vi "GS_Read_Config.vi"(4 "error in (no error)":errorcluster, 7 "Config Refnum":T1) -> (0 "error out":errorcluster, 2 "All Found?":bool, 3 "refnum out":T1)   [LabVIEW 2015]
uses:
  <vilib>/Utility/config.llb/Config Data RefNum.ctl
  <vilib>/Utility/config.llb/Read Key (Double).vi
  GSCS Scripting/Utils/GSP_Wavelength_Global.vi
  <vilib>/Utility/config.llb/NI_LVConfig.lvlib
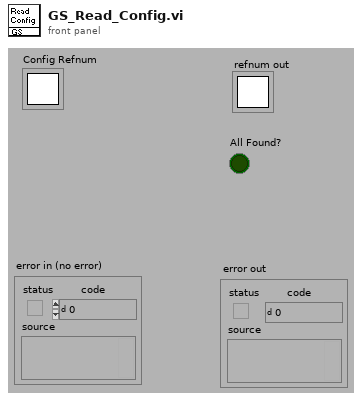
[diagram p1: front panel]
types:
  T1 = typedef "NI_LVConfig.lvlib/Config Data RefNum.ctl" = refnum<k1>
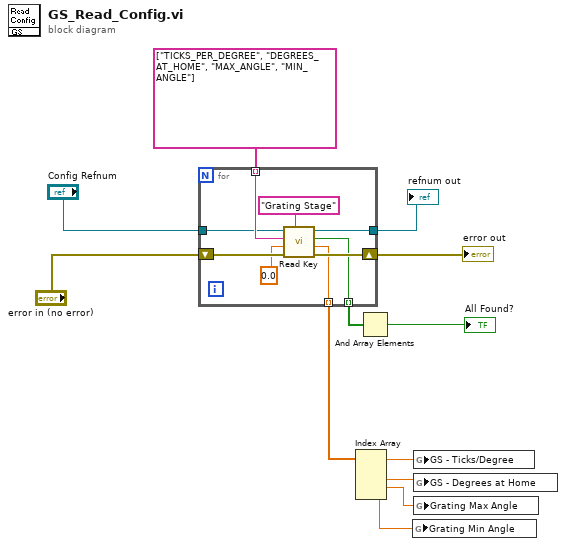
[diagram p0: block diagram]
diagram:
  n1 = for {
    shift-right: [w19] -> w11
    shift-left: "error in (no error)" -> [w21]
    tunnel: [w18] -> w12
    tunnel: string[] ["TICKS_PER_DEGREE", "DEGREES_AT_HOME", "MAX_ANGLE", "MIN_ANGLE"] -> [w17] mode=indexing
    tunnel: [w15] -> w10 mode=indexing
    tunnel: [w14] -> w9 mode=indexing
    tunnel: "Config Refnum" -> [w13]
    n2 = call-poly <vilib>:"Read Key.vi"("section"="Grating Stage", "error in (no error)"=w21, "default value"=0.0, "key"=w17, "refnum"=w13) -> ("error out"=w19:errorcluster, "value"=w15:dbl, "found?"=w14:bool, "refnum out"=w18:T1)  [unwired: 3 in]
  }
  "error out" <- w11
  "refnum out" <- w12
  n3 = Index Array(array=w10) -> (element #1=w3:dbl, element #2=w4:dbl, element #3=w2:dbl, element #4=w1:dbl)  [unwired: 4 in]
  n4 = And Array Elements(Boolean array=w9) -> (logical AND=→"All Found?":bool)
  n5 = global write "GSP_Wavelength_Global.vi" "Grating Min Angle"(w1) -> ()
  n6 = global write "GSP_Wavelength_Global.vi" "GS - Ticks/Degree"(w3) -> ()
  n7 = global write "GSP_Wavelength_Global.vi" "GS - Degrees at Home"(w4) -> ()
  n8 = global write "GSP_Wavelength_Global.vi" "Grating Max Angle"(w2) -> ()
